vi "parse.vi"(8 "error in (no error)":errorcluster, 10 "Message":u8[](array[numeric]) format="%02x", 11 "DLRS1ADisplacementGauge in":refnum<class "DLRS1ADisplacementGauge.lvclass">) -> (0 "error out":errorcluster, 2 "Error":bool, 3 "DLRS1ADisplacementGauge out":refnum<class "DLRS1ADisplacementGauge.lvclass">)   [LabVIEW 2016, in "RTDLRS1ADisplacementGauge.lvlib" / "DLRS1ADisplacementGauge.lvclass"]
uses:
  DLRS1ADisplacementGauge.lvclass
  DataTypes/DLRS1ADisplacementGaugeErrors.ctl
  DLRS1ADisplacementGauge.lvclass/DLRS1ADisplacementGauge.ctl
  RTDLRS1ADisplacementGauge.lvlib
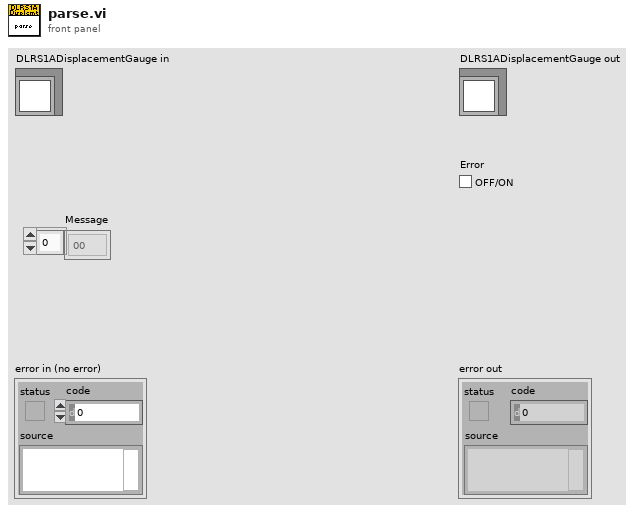
[diagram p1: front panel]
types:
  T1 = typedef "RTDLRS1ADisplacementGauge.lvlib/DLRS1ADisplacementGaugeErrors.ctl" = enum8{"None", "InvalidCommand", "CommunicationTimeoutError", "DataLengthError", "NumberOfParametersError", "ParameterError", "CommunicationError", "IDNumberError", "ExpansionLineError", "WriteControlError", "UnknownError", "UnknownResponseError"}
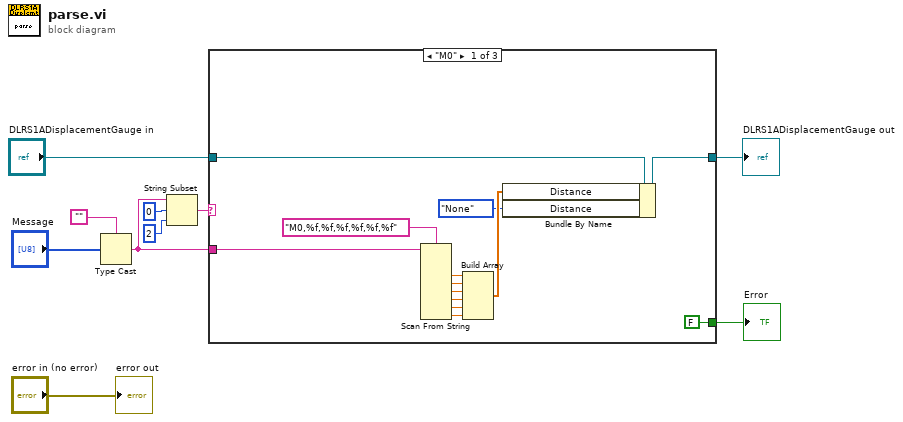
[diagram p0: block diagram]
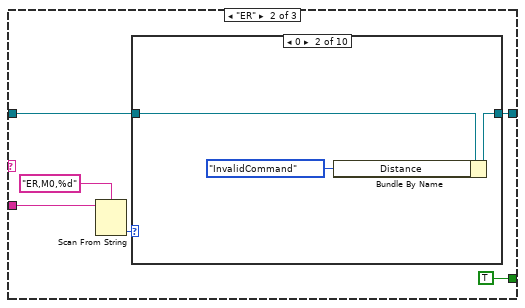
[diagram p2: hidden frame]
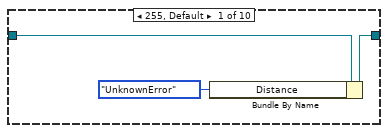
[diagram p3: hidden frame]
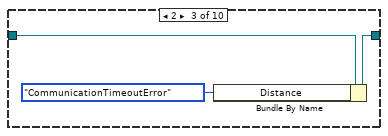
[diagram p4: hidden frame]
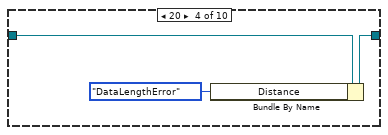
[diagram p5: hidden frame]
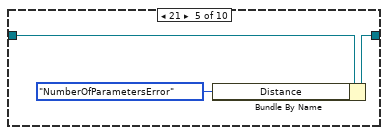
[diagram p6: hidden frame]
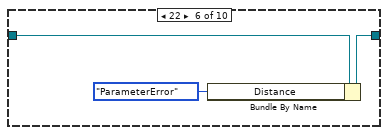
[diagram p7: hidden frame]
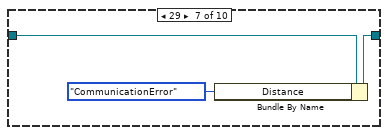
[diagram p8: hidden frame]
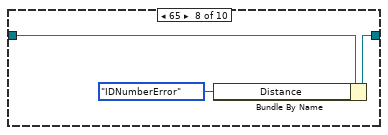
[diagram p9: hidden frame]
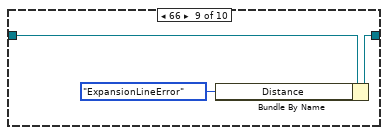
[diagram p10: hidden frame]
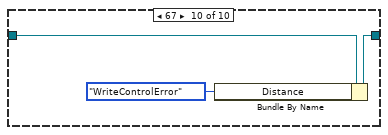
[diagram p11: hidden frame]
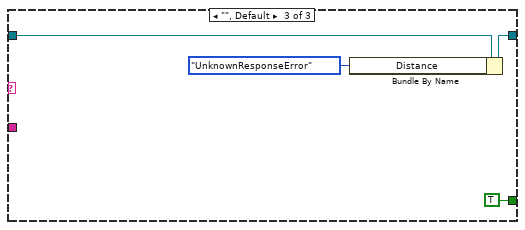
[diagram p12: hidden frame]
diagram:
  n1 = Type Cast(type="", x="Message") -> (*(type *) &x=w4:string)
  n2 = String Subset(string=w4, offset (0)=0, length (rest)=2 ("length (rest)")) -> (substring=w5:string)
  n3 = case shown="\"M0\"" w5 {
    tunnel: w4 -> [w22 w28 _]
    tunnel: "DLRS1ADisplacementGauge in" -> [w15 w26 w62]
    tunnel: [w14 w25 w61] -> w2
    tunnel: [FALSE TRUE TRUE] -> w1
    frame "M0" {
      n4 = Scan From String(format string="M0,%f,%f,%f,%f,%f,%f", input string=w22) -> (output 1=w21:dbl, output 2=w20:dbl, output 3=w19:dbl, output 4=w18:dbl, output 5=w17:dbl, output 6=w16:dbl)  [unwired: 8 in, 3 out]
      n5 = Build Array(w21, w20, w19, w18, w17, w16) -> (w13:dbl[])
      n6 = Bundle By Name(cluster=w15, "Distance"=w13, "Distance"=DLRS1ADisplacementGaugeErrors."None" ("Data.Responses.Distance")) -> (w14:refnum<class "DLRS1ADisplacementGauge.lvclass">)
    }
    frame "ER" {
      n7 = Scan From String(format string="ER,M0,%d", input string=w28) -> (output 1=w27:i32)  [unwired: 3 in, 3 out]
      n8 = case shown="0" w27 {
        tunnel: w26 -> [w32 w35 w38 w41 w44 w47 w50 w53 w56 w59]
        tunnel: [w31 w34 w37 w40 w43 w46 w49 w52 w55 w58] -> w25
        frame 255, Default {
          n9 = Bundle By Name(cluster=w32, "Distance"=DLRS1ADisplacementGaugeErrors."UnknownError" ("Data.Responses.Distance")) -> (w31:refnum<class "DLRS1ADisplacementGauge.lvclass">)
        }
        frame 0 {
          n10 = Bundle By Name(cluster=w35, "Distance"=DLRS1ADisplacementGaugeErrors."InvalidCommand" ("Data.Responses.Distance")) -> (w34:refnum<class "DLRS1ADisplacementGauge.lvclass">)
        }
        frame 2 {
          n11 = Bundle By Name(cluster=w38, "Distance"=DLRS1ADisplacementGaugeErrors."CommunicationTimeoutError" ("Data.Responses.Distance")) -> (w37:refnum<class "DLRS1ADisplacementGauge.lvclass">)
        }
        frame 20 {
          n12 = Bundle By Name(cluster=w41, "Distance"=DLRS1ADisplacementGaugeErrors."DataLengthError" ("Data.Responses.Distance")) -> (w40:refnum<class "DLRS1ADisplacementGauge.lvclass">)
        }
        frame 21 {
          n13 = Bundle By Name(cluster=w44, "Distance"=DLRS1ADisplacementGaugeErrors."NumberOfParametersError" ("Data.Responses.Distance")) -> (w43:refnum<class "DLRS1ADisplacementGauge.lvclass">)
        }
        frame 22 {
          n14 = Bundle By Name(cluster=w47, "Distance"=DLRS1ADisplacementGaugeErrors."ParameterError" ("Data.Responses.Distance")) -> (w46:refnum<class "DLRS1ADisplacementGauge.lvclass">)
        }
        frame 29 {
          n15 = Bundle By Name(cluster=w50, "Distance"=DLRS1ADisplacementGaugeErrors."CommunicationError" ("Data.Responses.Distance")) -> (w49:refnum<class "DLRS1ADisplacementGauge.lvclass">)
        }
        frame 65 {
          n16 = Bundle By Name(cluster=w53, "Distance"=DLRS1ADisplacementGaugeErrors."IDNumberError" ("Data.Responses.Distance")) -> (w52:refnum<class "DLRS1ADisplacementGauge.lvclass">)
        }
        frame 66 {
          n17 = Bundle By Name(cluster=w56, "Distance"=DLRS1ADisplacementGaugeErrors."ExpansionLineError" ("Data.Responses.Distance")) -> (w55:refnum<class "DLRS1ADisplacementGauge.lvclass">)
        }
        frame 67 {
          n18 = Bundle By Name(cluster=w59, "Distance"=DLRS1ADisplacementGaugeErrors."WriteControlError" ("Data.Responses.Distance")) -> (w58:refnum<class "DLRS1ADisplacementGauge.lvclass">)
        }
      }
    }
    frame "", Default {
      n19 = Bundle By Name(cluster=w62, "Distance"=DLRS1ADisplacementGaugeErrors."UnknownResponseError" ("Data.Responses.Distance")) -> (w61:refnum<class "DLRS1ADisplacementGauge.lvclass">)
    }
  }
  "DLRS1ADisplacementGauge out" <- w2
  "Error" <- w1
  "error out" <- "error in (no error)"
